vi "WaitPass2.vi"(8 "Best Y Inverso":dbl[](array[numeric]), 9 "Target":dbl[](array[numeric]), 10 "balls":T6[](array[typedef])=[{"x"=-2165.869384765625, "y"=510.4085693359375, "timestamp"=timestamp(2082758857.4639893 s since 1904-01-01), "Vel_x"=0.0, "Vel_y"=0.0, "Pos Bola Est"=[]}], 11 "Robot in":T1) -> (2 "Robot out":T1)   [LabVIEW 2017]
uses:
  Core/AI Robot.ctl
  Functions Enum.ctl
  AttackerStates.ctl
  Path Planning/RRT/PathDests.ctl
  Path Planning/RRT/PathDest.ctl
  Core/AI Ball.ctl
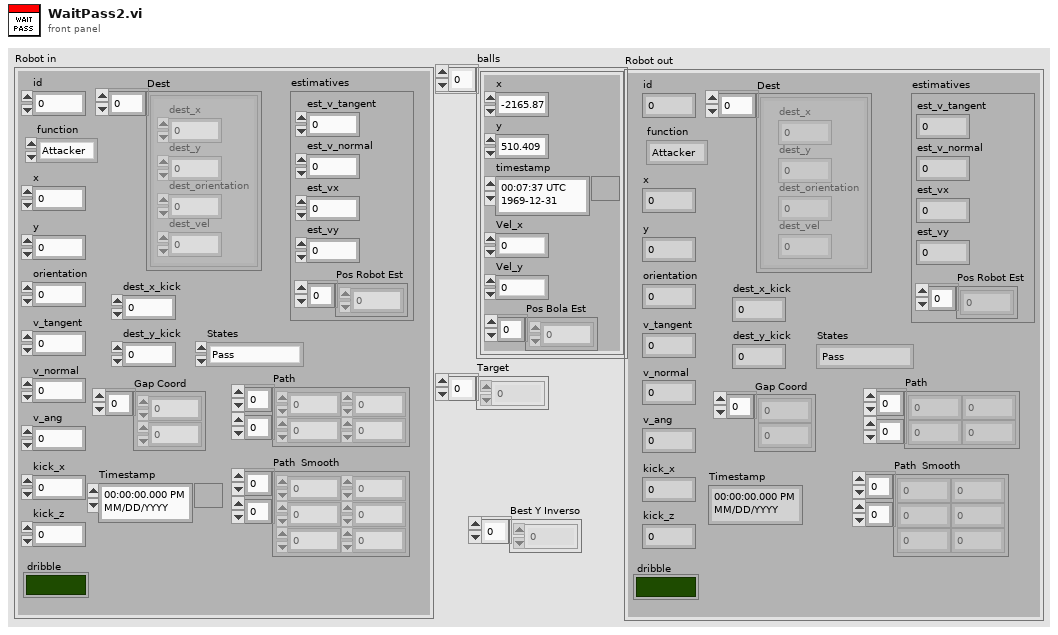
[diagram p1: front panel]
types:
  T1 = typedef "AI Robot.ctl" = cluster{"id":u32, "function":T2, "x":dbl, "y":dbl, "orientation":dbl, "v_tangent":dbl, "v_normal":dbl, "v_ang":dbl, "kick_x":dbl, "kick_z":dbl, "dribble":bool, "Timestamp":timestamp, "estimatives":cluster{"est_v_tangent":dbl, "est_v_normal":dbl, "est_vx":dbl, "est_vy":dbl, "Pos Robot Est":dbl[]}, "dest_x_kick":dbl, "dest_y_kick":dbl, "Gap Coord":dbl[], "States":T3, "Path ":dbl[][], "Path  Smooth":dbl[][], "Dest":T4}
  T2 = typedef "Functions Enum.ctl" = enum16{"Attacker", "Goalie", "Defender", "Striker", "Goto 0", "Dummy", "Kicker", "ZigZag"}
  T3 = typedef "AttackerStates.ctl" = enum16{"Pass", "GoToTangent", "BallGetting", "GoToKick", ""}
  T4 = typedef "PathDests.ctl" = T5[]
  T5 = typedef "PathDest.ctl" = cluster{"dest_x":dbl, "dest_y":dbl, "dest_orientation":dbl, "dest_vel":dbl}
  T6 = typedef "AI Ball.ctl" = cluster{"x":dbl, "y":dbl, "timestamp":timestamp, "Vel_x":dbl, "Vel_y":dbl, "Pos Bola Est":dbl[]}
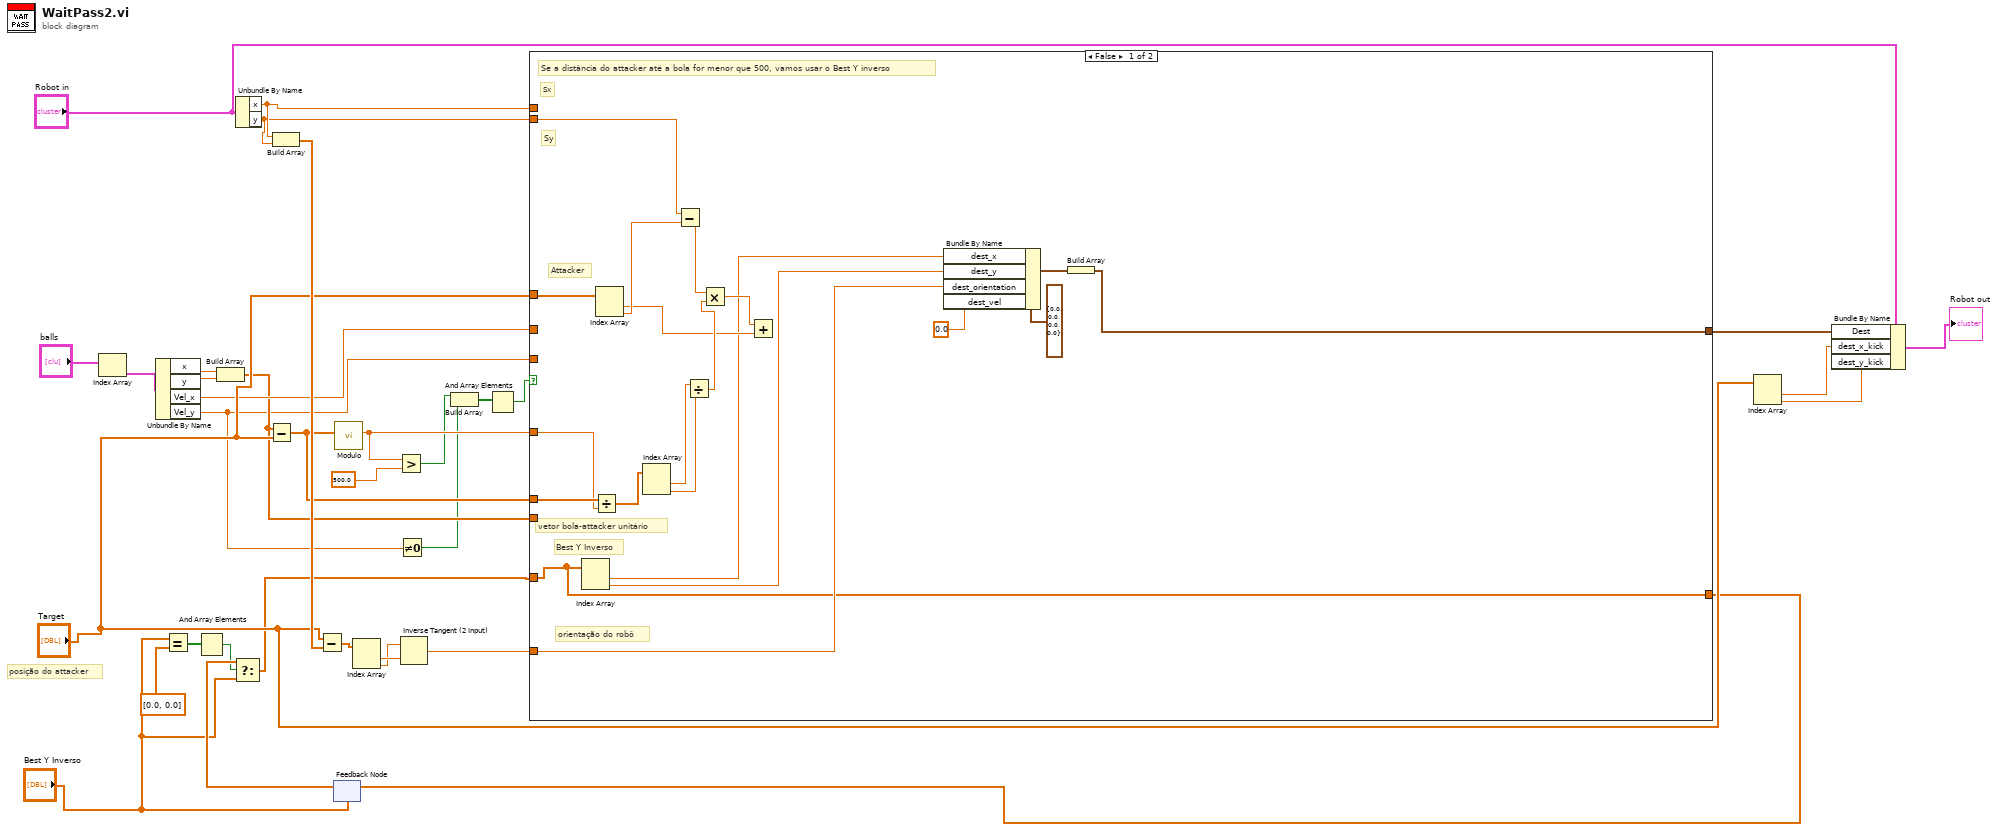
[diagram p0: block diagram]
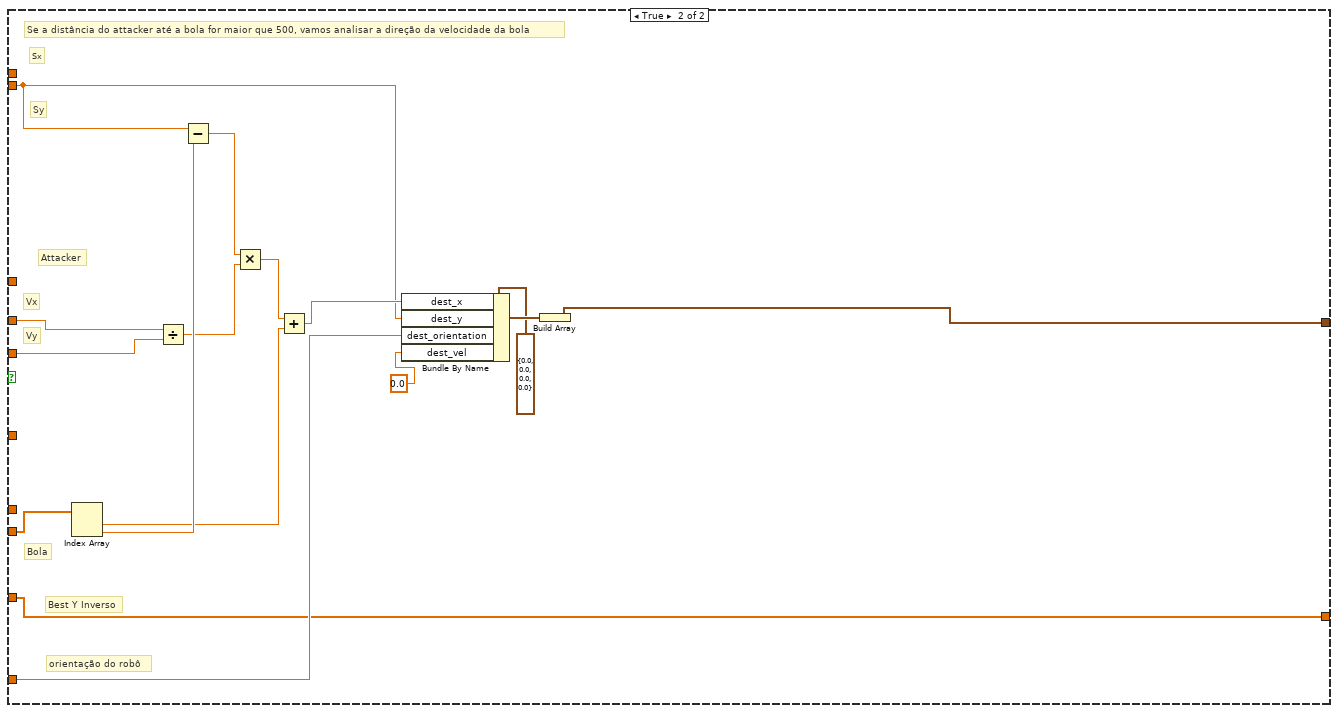
[diagram p2: hidden frame]
diagram:
  # "posição do attacker"
  n1 = Index Array(array="balls") -> (element=w33:T6)  [unwired: 1 in]
  n2 = Unbundle By Name(w33) -> ("x"=w32:dbl, "y"=w31:dbl, "Vel_x"=w16:dbl, "Vel_y"=w11:dbl)
  n3 = Equal?(x="Best Y Inverso", y=dbl[] [0.0, 0.0] ("FinalPosition")) -> (x = y?=w2:bool[])
  n4 = And Array Elements(Boolean array=w2) -> (logical AND=w1:bool)
  n5 = Build Array(w32, w31) -> (w15:dbl[])
  n6 = Unbundle By Name("Robot in") -> ("x"=w25:dbl, "y"=w24:dbl)
  n7 = Subtract(x=w15, y="Target") -> (x-y=w14:dbl[])
  n8 = Build Array(w25, w24) -> (w23:dbl[])
  n9 = Subtract(x="Target", y=w23) -> (x-y=w26:dbl[])
  n10 = feedback #1("Best Y Inverso") -> (w5:dbl[])
  n11 = Select(t=w5, s=w1, f="Best Y Inverso") -> (s? t:f=w4:dbl[])
  n12 = call "Modulo.vi"("2D vector"=w14) -> ("Modulo"=w29:dbl)  [unwired: 10 in]
  n13 = Index Array(array=w26) -> (element #1=w28:dbl, element #2=w27:dbl)  [unwired: 2 in]
  n14 = Greater?(x=w29, y=500.0) -> (0:w13:bool)
  n15 = Not Equal To 0?(x=w11) -> (x != 0?=w12:bool)
  n16 = Inverse Tangent (2 Input)(1:w28, 2:w27) -> (0:w22:dbl)
  n17 = Build Array(w13, w12) -> (w10:bool[])
  n18 = And Array Elements(Boolean array=w10) -> (logical AND=w9:bool)
  n19 = case shown="False" w9 {
    tunnel: w25 -> [_ _]
    tunnel: w24 -> [w40 w56]
    tunnel: w14 -> [w54 _]
    tunnel: w29 -> [w53 _]
    tunnel: "Target" -> [w51 _]
    tunnel: w22 -> [w39 w59]
    tunnel: [w38 w58] -> w20
    tunnel: w16 -> [_ w70]
    tunnel: w11 -> [_ w69]
    tunnel: w15 -> [_ w68]
    tunnel: w4 -> [w35 w55]
    tunnel: [w35 w55] -> w7
    frame False {
      # "Best Y Inverso"
      # "Se a distância do attacker até a bola for menor que 500, vamos usar o Best Y inverso"
      # "orientação do robô"
      # "Attacker"
      # "Sy"
      # "Sx"
      # "vetor bola-attacker unitário"
      n20 = Index Array(array=w35) -> (element #1=w37:dbl, element #2=w36:dbl)  [unwired: 2 in]
      n21 = Divide(x=w54, y=w53) -> (x/y=w52:dbl[])
      n22 = Index Array(array=w51) -> (element #1=w44:dbl, element #2=w50:dbl)  [unwired: 2 in]
      n23 = Index Array(array=w52) -> (element #1=w49:dbl, element #2=w48:dbl)  [unwired: 2 in]
      n24 = Subtract(x=w40, y=w50) -> (x-y=w47:dbl)
      n25 = Divide(x=w49, y=w48) -> (x/y=w46:dbl)
      n26 = Multiply(x=w47, y=w46) -> (x*y=w45:dbl)
      n27 = Add(x=w45, y=w44) -> ()  [unwired: 1 out]
      n28 = Bundle By Name(cluster=T5 {"dest_x"=0.0, "dest_y"=0.0, "dest_orientation"=0.0, "dest_vel"=0.0} ("Dest"), "dest_x"=w37, "dest_y"=w36, "dest_orientation"=w39, "dest_vel"=0.0) -> (w42:T5)
      n29 = Build Array(w42) -> (w38:T5[])
    }
    frame True {
      # "Best Y Inverso"
      # "Bola"
      # "Vy"
      # "Vx"
      # "orientação do robô"
      # "Attacker"
      # "Sy"
      # "Sx"
      # "Se a distância do attacker até a bola for maior que 500, vamos analisar a direção da velocidade da bola"
      n30 = Index Array(array=w68) -> (element #1=w63:dbl, element #2=w67:dbl)  [unwired: 2 in]
      n31 = Divide(x=w70, y=w69) -> (x/y=w65:dbl)
      n32 = Subtract(x=w56, y=w67) -> (x-y=w66:dbl)
      n33 = Multiply(x=w66, y=w65) -> (x*y=w64:dbl)
      n34 = Add(x=w64, y=w63) -> (x+y=w57:dbl)
      n35 = Bundle By Name(cluster=T5 {"dest_x"=0.0, "dest_y"=0.0, "dest_orientation"=0.0, "dest_vel"=0.0} ("Dest"), "dest_x"=w57, "dest_y"=w56, "dest_orientation"=w59, "dest_vel"=0.0) -> (w62:T5)
      n36 = Build Array(w62) -> (w58:T5[])
    }
  }
  n37 = feedback-in #1(w7) -> ()
  n38 = Index Array(array="Target") -> (element #1=w19:dbl, element #2=w18:dbl)  [unwired: 2 in]
  n39 = Bundle By Name(cluster="Robot in", "Dest"=w20, "dest_x_kick"=w19, "dest_y_kick"=w18) -> (→"Robot out":T1)
